vi "SetClassCluster.vi"(8 "error in (no error)":errorcluster, 11 "Experiment.lvclass":refnum<class "Experiment.lvclass">) -> (0 "error out":errorcluster, 2 "Experiment Data":T1, 3 "Experiment.lvclass Out":refnum<class "Experiment.lvclass">)   [LabVIEW 2019, in "Experiment.lvclass"]
uses:
  Experiment.lvclass
  ClassCluster.ctl
  DevicesClass/BaseDevice/BaseDevice.lvclass
  Experiment.lvclass/Experiment.ctl
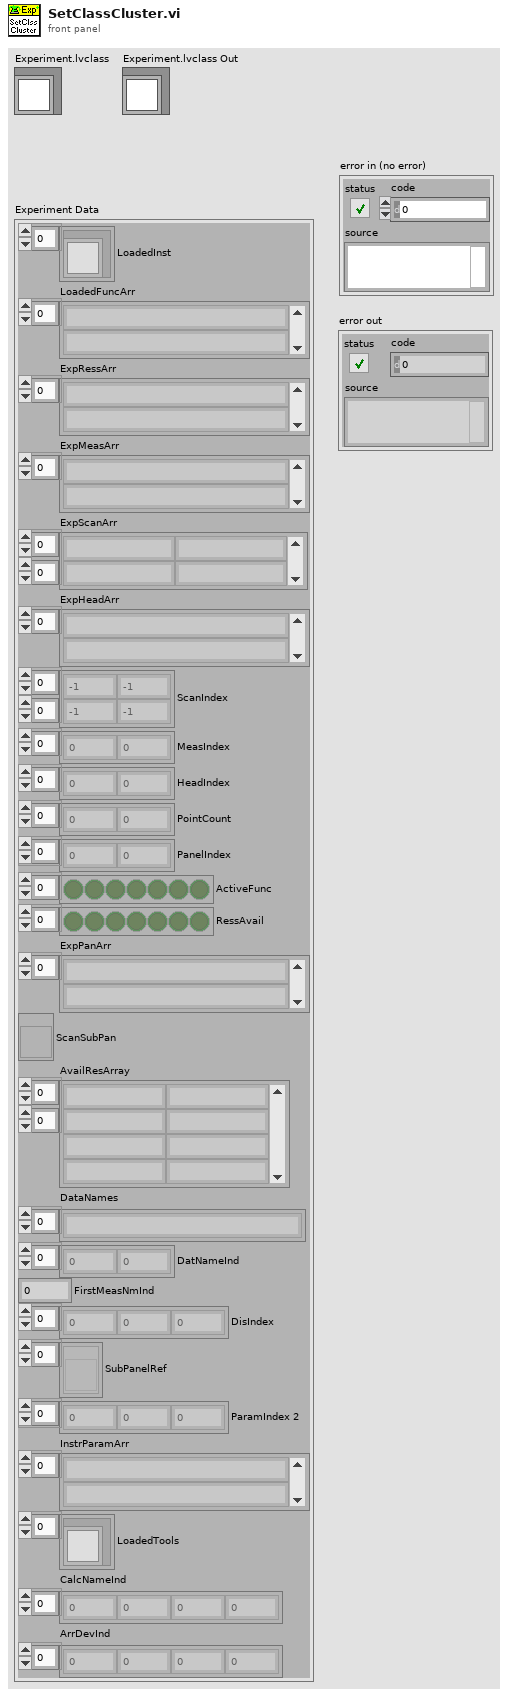
[diagram p1: front panel]
types:
  T1 = typedef "ClassCluster.ctl" = cluster{"LoadedInst":refnum<class "BaseDevice.lvclass">[], "LoadedFuncArr":string[], "ExpRessArr":string[], "ExpMeasArr":string[], "ExpScanArr":string[][], "ExpHeadArr":string[], "ScanIndex":i32[][], "MeasIndex":i32[], "HeadIndex":i32[], "PointCount":i32[], "PanelIndex":i32[], "ActiveFunc":bool[], "RessAvail":bool[], "ExpPanArr":string[], "ScanSubPan":refnum<vi>, "AvailResArray":string[][], "DataNames":string[], "DatNameInd":i32[], "FirstMeasNmInd":i32, "DisIndex":i32[], "SubPanelRef":refnum<vi>[], "ParamIndex 2":i32[], "InstrParamArr":string[], "LoadedTools":refnum<class "BaseDevice.lvclass">[], "CalcNameInd":i32[], "ArrDevInd":i32[]}
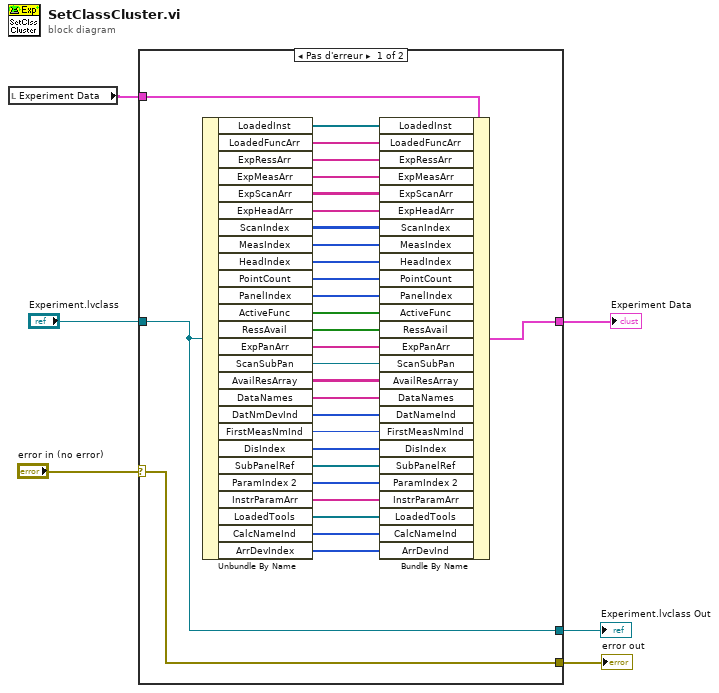
[diagram p0: block diagram]
diagram:
  n1 = local read "Experiment Data"() -> (w1:T1)
  n2 = case shown="Pas d'erreur" "error in (no error)" {
    selector: "error in (no error)" -> [w12 w38]
    tunnel: "Experiment.lvclass" -> [w11 w39]
    tunnel: [w9 w37] -> w5
    tunnel: [w12 w38] -> w3
    tunnel: [w11 w39] -> w2
    tunnel: w1 -> [w10 w37]
    frame No Error {
      n3 = Unbundle By Name(w11) -> ("LoadedInst"=w36:refnum<class "BaseDevice.lvclass">[], "LoadedFuncArr"=w35:string[], "ExpRessArr"=w34:string[], "ExpMeasArr"=w33:string[], "ExpScanArr"=w32:string[][], "ExpHeadArr"=w31:string[], "ScanIndex"=w30:i32[][], "MeasIndex"=w29:i32[], "HeadIndex"=w28:i32[], "PointCount"=w27:i32[], "PanelIndex"=w26:i32[], "ActiveFunc"=w25:bool[], "RessAvail"=w24:bool[], "ExpPanArr"=w23:string[], "ScanSubPan"=w22:refnum<vi>, "AvailResArray"=w21:string[][], "DataNames"=w20:string[], "DatNmDevInd"=w19:i32[], "FirstMeasNmInd"=w18:i32, "DisIndex"=w17:i32[], "SubPanelRef"=w16:refnum<vi>[], "ParamIndex 2"=w15:i32[], "InstrParamArr"=w14:string[], "LoadedTools"=w13:refnum<class "BaseDevice.lvclass">[], "CalcNameInd"=w8:i32[], "ArrDevIndex"=w7:i32[])
      n4 = Bundle By Name(cluster=w10, "LoadedInst"=w36, "LoadedFuncArr"=w35, "ExpRessArr"=w34, "ExpMeasArr"=w33, "ExpScanArr"=w32, "ExpHeadArr"=w31, "ScanIndex"=w30, "MeasIndex"=w29, "HeadIndex"=w28, "PointCount"=w27, "PanelIndex"=w26, "ActiveFunc"=w25, "RessAvail"=w24, "ExpPanArr"=w23, "ScanSubPan"=w22, "AvailResArray"=w21, "DataNames"=w20, "DatNameInd"=w19, "FirstMeasNmInd"=w18, "DisIndex"=w17, "SubPanelRef"=w16, "ParamIndex 2"=w15, "InstrParamArr"=w14, "LoadedTools"=w13, "CalcNameInd"=w8, "ArrDevInd"=w7) -> (w9:T1)
    }
    frame Error {
    }
  }
  "Experiment Data" <- w5
  "Experiment.lvclass Out" <- w2
  "error out" <- w3
